vi "Layout.vi"(0 "FSM.Edge In":refnum<class "FSM.Edge.lvclass">) -> (4 "FSM.Edge Out":refnum<class "FSM.Edge.lvclass">)   [LabVIEW 2020, in "FSM.Edge.lvclass"]
uses:
  FSM.Edge.lvclass
  FSM.Edge.lvclass/FSM.Edge.ctl
  FSM.Label/FSM.Label.lvclass
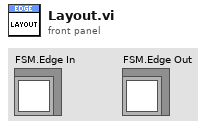
[diagram p1: front panel]
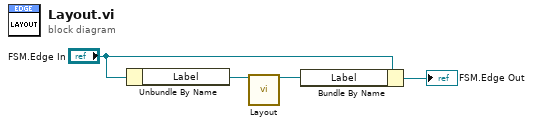
[diagram p0: block diagram]
diagram:
  n1 = Unbundle By Name("FSM.Edge In") -> ("Label"=w4:refnum<class "FSM.Label.lvclass">)
  n2 = call "Layout.vi"("FSM.Label In"=w4) -> ("FSM.Label Out"=w2:refnum<class "FSM.Label.lvclass">)  [unwired: 14 in]
  n3 = Bundle By Name(cluster="FSM.Edge In", "Label"=w2) -> (→"FSM.Edge Out":refnum<class "FSM.Edge.lvclass">)
